vi "Configure Servo.vi"(8 "error in":errorcluster, 11 "tCRD in":refnum<class "Aircraft OPCCRD.lvclass">) -> (0 "error out":errorcluster, 3 "tCRD out":refnum<class "Aircraft OPCCRD.lvclass">)   [LabVIEW 2015, in "Aircraft OPCCRD.lvclass"]
uses:
  Aircraft OPCCRD.lvclass
  Switch/Servo Switch.lvclass
  <vilib>/Utility/config.llb/NI_LVConfig.lvlib
  <vilib>/Utility/config.llb/Read Key (Double).vi
  <vilib>/Utility/config.llb/Read Key (Boolean).vi
  <vilib>/Utility/config.llb/Read Key (I32).vi
  Reusable/Session APIs/File Access/Config Data/Config Data.lvclass
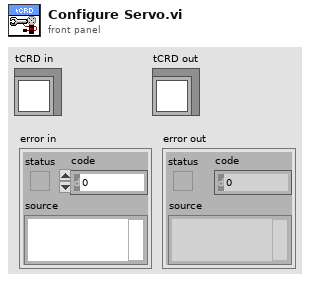
[diagram p1: front panel]
types:
  T1 = typedef "Config Data.lvclass/Config Session.ctl" = refnum<data-value>
  T2 = typedef "NI_LVConfig.lvlib/Config Data RefNum.ctl" = refnum<k1>
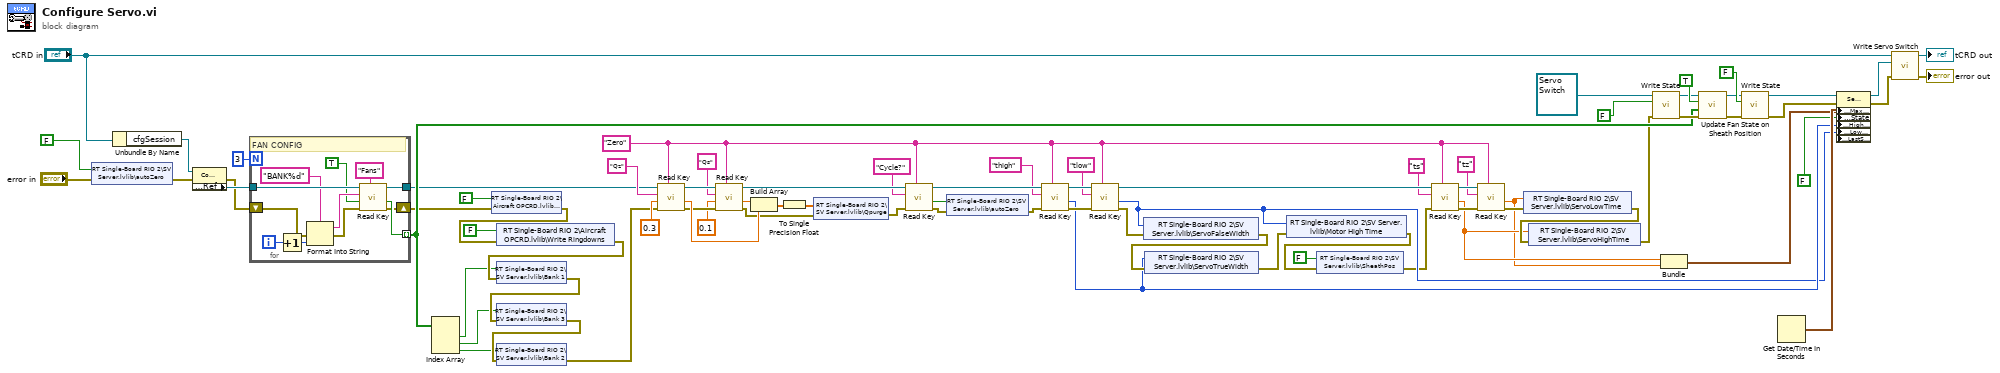
[diagram p0: block diagram]
diagram:
  w42 = "Zero" ("section")
  n1 = shared-variable "RT Single-Board RIO 2\\SV Server.lvlib\\autoZero"(FALSE ("autoZero"), error in="error in") -> (error out=w28:errorcluster)
  n2 = Unbundle By Name("tCRD in") -> ("cfgSession"=w69:T1)
  n3 = property class="Config Data"(reference=w69, error in=w28) -> (error out=w6:errorcluster, "Accessors:Ref"=w8:T2)  [unwired: 1 out]
  n4 = for {
    N: 3 -> [_]
    tunnel: w8 -> [w91]
    tunnel: [w85] -> w10 mode=indexing
    tunnel: [w83] -> w7
    shift-right: [w81] -> w4
    shift-left: w6 -> [w80]
    i -> [w89]
    # "FAN CONFIG"
    n5 = Increment(x=w89) -> (x+1=w88:i32)
    n6 = Format Into String(format string="BANK%d", error in=w80, w88) -> (resulting string=w86:string, error out=w82:errorcluster)  [unwired: 1 in]
    n7 = call-poly <vilib>:"Read Key.vi"("section"="Fans", "error in (no error)"=w82, "default value"=TRUE, "key"=w86, "refnum"=w91) -> ("error out"=w81:errorcluster, "value"=w85:bool, "refnum out"=w83:T2)  [unwired: 3 in, 1 out]
  }
  n8 = Index Array(array=w10) -> (element #1=w20:bool, element #2=w19:bool, element #3=w18:bool)  [unwired: 3 in]
  n9 = shared-variable "RT Single-Board RIO 2\\Aircraft OPCRD.lvlib\\Invert?"(FALSE ("Invert?"), error in=w4) -> (error out=w5:errorcluster)
  n10 = shared-variable "RT Single-Board RIO 2\\Aircraft OPCRD.lvlib\\Write Ringdowns"(FALSE ("Write Ringdowns"), error in=w5) -> (error out=w24:errorcluster)
  n11 = shared-variable "RT Single-Board RIO 2\\SV Server.lvlib\\Bank 1"(w20, error in=w24) -> (error out=w23:errorcluster)
  n12 = shared-variable "RT Single-Board RIO 2\\SV Server.lvlib\\Bank 3"(w19, error in=w23) -> (error out=w22:errorcluster)
  n13 = shared-variable "RT Single-Board RIO 2\\SV Server.lvlib\\Bank 2"(w18, error in=w22) -> (error out=w3:errorcluster)
  n14 = call-poly <vilib>:"Read Key.vi"("section"=w42, "error in (no error)"=w3, "default value"=0.3, "key"="Qz", "refnum"=w7) -> ("error out"=w63:errorcluster, "value"=w64:dbl, "refnum out"=w68:T2)  [unwired: 3 in, 1 out]
  n15 = call-poly <vilib>:"Read Key.vi"("section"=w42, "error in (no error)"=w63, "default value"=0.1, "key"="Qs", "refnum"=w68) -> ("error out"=w62:errorcluster, "value"=w65:dbl, "refnum out"=w59:T2)  [unwired: 3 in, 1 out]
  n16 = Build Array(w65, w64) -> (w61:dbl[])
  n17 = To Single Precision Float(number=w61) -> (single precision float=w60:sgl[])
  n18 = shared-variable "RT Single-Board RIO 2\\SV Server.lvlib\\Qpurge"(w60, error in=w62) -> (error out=w58:errorcluster)
  n19 = call-poly <vilib>:"Read Key.vi"("section"=w42, "error in (no error)"=w58, "key"="Cycle?", "refnum"=w59) -> ("error out"=w55:errorcluster, "value"=w56:bool, "refnum out"=w54:T2)  [unwired: 4 in, 1 out]
  n20 = shared-variable "RT Single-Board RIO 2\\SV Server.lvlib\\autoZero"(w56, error in=w55) -> (error out=w53:errorcluster)
  n21 = call-poly <vilib>:"Read Key.vi"("section"=w42, "error in (no error)"=w53, "key"="thigh", "refnum"=w54) -> ("error out"=w51:errorcluster, "value"=w37:i32, "refnum out"=w52:T2)  [unwired: 4 in, 1 out]
  n22 = call-poly <vilib>:"Read Key.vi"("section"=w42, "error in (no error)"=w51, "key"="tlow", "refnum"=w52) -> ("error out"=w47:errorcluster, "value"=w36:i32, "refnum out"=w48:T2)  [unwired: 4 in, 1 out]
  n23 = shared-variable "RT Single-Board RIO 2\\SV Server.lvlib\\ServoFalseWidth"(w36, error in=w47) -> (error out=w45:errorcluster)
  n24 = shared-variable "RT Single-Board RIO 2\\SV Server.lvlib\\ServoTrueWidth"(w37, error in=w45) -> (error out=w32:errorcluster)
  n25 = shared-variable "RT Single-Board RIO 2\\SV Server.lvlib\\Motor High Time"(w36, error in=w32) -> (error out=w31:errorcluster)
  n26 = shared-variable "RT Single-Board RIO 2\\SV Server.lvlib\\SheathPos"(FALSE ("SheathPos"), error in=w31) -> (error out=w30:errorcluster)
  n27 = call-poly <vilib>:"Read Key.vi"("section"=w42, "error in (no error)"=w30, "key"="ts", "refnum"=w48) -> ("error out"=w43:errorcluster, "value"=w35:dbl, "refnum out"=w44:T2)  [unwired: 4 in, 1 out]
  n28 = call-poly <vilib>:"Read Key.vi"("section"=w42, "error in (no error)"=w43, "key"="tz", "refnum"=w44) -> ("error out"=w40:errorcluster, "value"=w34:dbl)  [unwired: 4 in, 2 out]
  n29 = shared-variable "RT Single-Board RIO 2\\SV Server.lvlib\\ServoLowTime"(w34, error in=w40) -> (error out=w39:errorcluster)
  n30 = shared-variable "RT Single-Board RIO 2\\SV Server.lvlib\\ServoHighTime"(w35, error in=w39) -> (error out=w2:errorcluster)
  n31 = call-dynamic "Write State.vi"("error in"=w2, "State"=FALSE ("SheathPos"), "Switch in"=refnum<class "Servo Switch.lvclass"> refnum ("Servo Switch in")) -> ("error out"=w11:errorcluster, "Switch out"=w13:refnum<class "Servo Switch.lvclass">)  [unwired: 7 in]
  n32 = Bundle("value"=w35, "value"=w34) -> (w33:cluster{"value":dbl, "value":dbl})  [unwired: 1 in]
  n33 = call "Update Fan State on Sheath Position.vi"("error in"=w11, "Init Fan Pos"=w10, "Init?"=TRUE, "Servo Switch in"=w13) -> ("error out"=w1:errorcluster, "Servo Switch out"=w9:refnum<class "Servo Switch.lvclass">)  [unwired: 6 in]
  n34 = call-dynamic "Write State.vi"("error in"=w1, "State"=FALSE ("SheathPos"), "Switch in"=w9) -> ("error out"=w77:errorcluster, "Switch out"=w76:refnum<class "Servo Switch.lvclass">)  [unwired: 7 in]
  n35 = Get Date/Time In Seconds() -> (seconds since 1Jan1904=w79:timestamp)
  n36 = property class="Servo Switch"(reference=w76, error in=w77, "Data Access:Max Elapsed Time"=w33, "Data Access:State"=FALSE ("State"), "Accessors:High Time"=w37, "Accessors:Low Time"=w36, "Accessors:LastSwitch"=w79) -> (reference out=w74:refnum<class "Servo Switch.lvclass">, error out=w71:errorcluster)
  n37 = call "Write Servo Switch.vi"("error in (no error)"=w71, "Servo Switch"=w74, "tCRD in"="tCRD in") -> ("error out"=→"error out":errorcluster, "tCRD out"=→"tCRD out":refnum<class "Aircraft OPCCRD.lvclass">)  [unwired: 7 in]
